vi "niScope Multi Fetch Array Measurement Cluster.vi"(0 "instrument handle":refnum<k15>, 1 "timeout":dbl=5.0 format="%.2f", 5 "channels":string="0", 7 "array measurement":T3=4000 items=["None"=4000, "Last Acq. Histogram"=4001, "Multi Acq. Voltage Histogram"=4004, "Multi Acq. Time Histogram"=4005, "Multi Acq. Average"=4016, "Polynomial Interpolation"=4011, "Array Integral"=4006, "Derivative"=4007, "Inverse"=4008, "Multiply Channels"=4012, "Add Channels"=4013, "Subtract Channels"=4014, "Divide Channels"=4015, "Array Offset"=4025, "Array Gain"=4026, "Hanning Window"=4009, "Flat Top Window"=4010, "Hamming Window"=4020, "Triangle Window"=4023, "Blackman Window"=4024, "FIR Windowed Filter"=4021, "Bessel IIR Filter"=4022, "Butterworth IIR Filter"=4017, "Chebyshev IIR Filter"=4018, "FFT Phase Spectrum"=4002, "FFT Amp. Spectrum (Volts RMS)"=4003, "FFT Amp. Spectrum (dB)"=4019], 11 "error in":errorcluster, 12 "meas waveform size":i32=-1) -> (4 "instrument handle out":refnum<k15>, 6 "wfm info":T1(array[cluster]) {"reserved2" format="%.2f"; "reserved1" format="%.2f"; "offset" format="%^.3e"; "gain" format="%^.3e"; "xIncrement" format="%^.3e"; "relativeInitialX" format="%^.3e"; "absoluteInitialX" format="%^.3e"}, 10 "meas waveform":T2(array[cluster]) {"measWfm" format="%.2f"; "xIncrement" format="%.2f"; "relativeInitialX" format="%.2f"}, 15 "error out":errorcluster)   [LabVIEW 2011]
doc: "Obtains a waveform from the digitizer and returns the specified array measurement for multiple channels and records as a cluster."
uses:
  <instrlib>/niScope/Controls/niScope array measurement.ctl
  niScope_32.dll
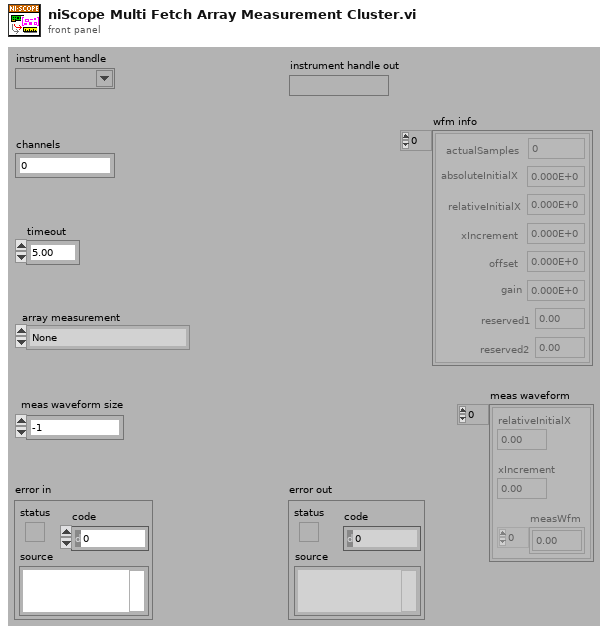
[diagram p1: front panel]
types:
  T1 = cluster{"actualSamples":i32, "absoluteInitialX":dbl, "relativeInitialX":dbl, "xIncrement":dbl, "offset":dbl, "gain":dbl, "reserved1":dbl, "reserved2":dbl}[]
  T2 = cluster{"relativeInitialX":dbl, "xIncrement":dbl, "measWfm":dbl[]}[]
  T3 = typedef "niScope array measurement.ctl" = i32
  T4 = cluster{"Element Data":i32, "Element Data":dbl, "Element Data":dbl, "Element Data":dbl, "Element Data":dbl, "Element Data":dbl, "Element Data":dbl, "Element Data":dbl}
  T5 = cluster{"Element Data":dbl, "Element Data":dbl, "measWfm":dbl[]}
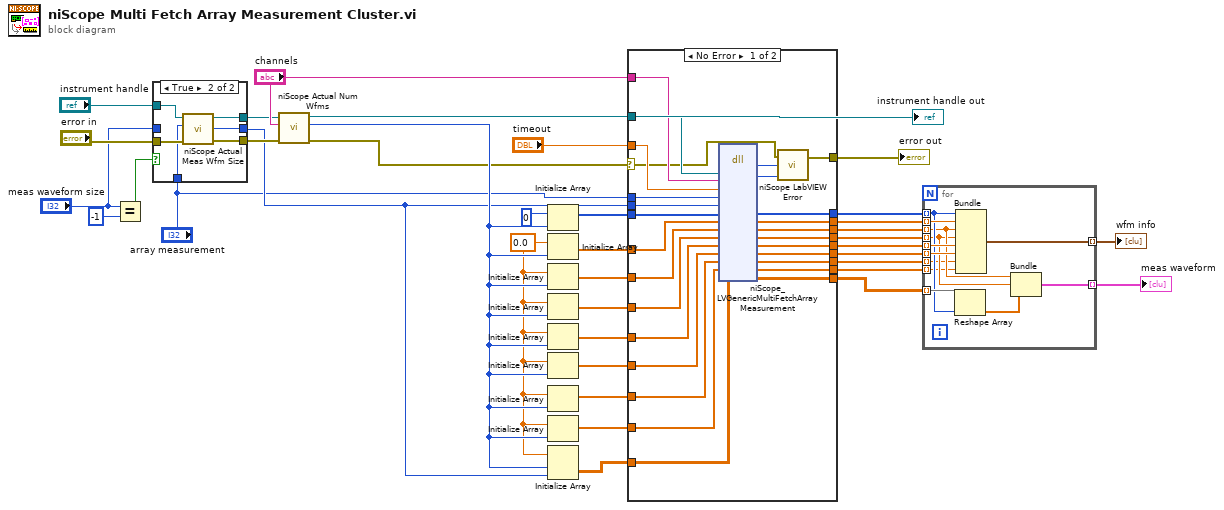
[diagram p0: block diagram]
diagram:
  w8 = 0.0 ("Element Data")
  n1 = Equal?(x="meas waveform size", y=-1) -> (x = y?=w34:bool)
  n2 = case shown="True" w34 {
    tunnel: [w40 w46] -> w33
    tunnel: "error in" -> [w40 w45]
    tunnel: "instrument handle" -> [w39 w44]
    tunnel: [w39 w43] -> w30
    tunnel: [w38 w42] -> w27
    tunnel: "meas waveform size" -> [w38 _]
    tunnel: "array measurement" -> [_ w41]
    frame False {
    }
    frame True {
      n3 = call <instrlib>:"niScope Actual Meas Wfm Size.vi"("error in"=w45, "arrayMeasFunction"=w41, "instrument handle"=w44) -> ("error out"=w46:errorcluster, "meas wfm size"=w42:i32, "instrument handle out"=w43:refnum<k15>)  [unwired: 6 in]
    }
  }
  n4 = call <instrlib>:"niScope Actual Num Wfms.vi"("error in"=w33, "channels"="channels", "instrument handle"=w30) -> ("error out"=w1:errorcluster, "actual num wfms"=w28:i32, "instrument handle out"=w26:refnum<k15>)  [unwired: 6 in]
  "instrument handle out" <- w26
  n5 = Initialize Array(0 ("Element Data"), w28) -> (w18:i32[])
  n6 = Initialize Array(w8, w28) -> (w19:dbl[])
  n7 = Initialize Array(w8, w28) -> (w2:dbl[])
  n8 = Initialize Array(w8, w28) -> (w20:dbl[])
  n9 = Initialize Array(w8, w28) -> (w21:dbl[])
  n10 = Initialize Array(w8, w28) -> (w9:dbl[])
  n11 = Initialize Array(w8, w28) -> (w7:dbl[])
  n12 = Initialize Array(w8, w28) -> (w6:dbl[])
  n13 = Initialize Array(w8, w28, w27) -> (w10:dbl[][])
  n14 = case shown="No Error" w1 {
    selector: w1 -> [w47 w74]
    tunnel: [w73 w74] -> w37
    tunnel: "channels" -> [w72 _]
    tunnel: w27 -> [w71 _]
    tunnel: w26 -> [w70 _]
    tunnel: "array measurement" -> [w69 _]
    tunnel: w21 -> [w66 w79]
    tunnel: w20 -> [w65 w80]
    tunnel: w2 -> [w64 w81]
    tunnel: w19 -> [w63 w82]
    tunnel: w18 -> [w62 w83]
    tunnel: "timeout" -> [w61 _]
    tunnel: [w60 w78] -> w16
    tunnel: [w59 w79] -> w15
    tunnel: [w58 w80] -> w14
    tunnel: [w57 w81] -> w13
    tunnel: [w56 w82] -> w12
    tunnel: [w55 w83] -> w11
    tunnel: w10 -> [w54 w75]
    tunnel: w9 -> [w53 w78]
    tunnel: w7 -> [w52 w77]
    tunnel: w6 -> [w51 w76]
    tunnel: [w50 w75] -> w5
    tunnel: [w49 w77] -> w4
    tunnel: [w48 w76] -> w3
    frame No Error {
      n15 = dll-call lib="niScope_*.*" fn="niScope_LVGenericMultiFetchArrayMeasurement"("instrument handle"=w70, "channelList"=w72, "timeout"=w61, "arrayMeasFunction"=w69, "measWfmSize"=w71, "actualSamples"=w62, "absoluteInitialX"=w63, "relativeInitialX"=w64, "xIncrement"=w65, "offset"=w66, "gain"=w53, "reserved1"=w52, "reserved2"=w51, "measWfm"=w54) -> ("status"=w68:i32, "instrument handle"=w67:u32, "actualSamples"=w55:i32[], "absoluteInitialX"=w56:dbl[], "relativeInitialX"=w57:dbl[], "xIncrement"=w58:dbl[], "offset"=w59:dbl[], "gain"=w60:dbl[], "reserved1"=w49:dbl[], "reserved2"=w48:dbl[], "measWfm"=w50:dbl[][])  [unwired: 7 in, 2 out]
      n16 = call <instrlib>:"niScope LabVIEW Error.vi"("instrument handle"=w67, "niScope error code (0)"=w68, "error in (no error)"=w47) -> ("error out"=w73:errorcluster)  [unwired: 2 in]
    }
    frame Error {
    }
  }
  "error out" <- w37
  n17 = for {
    tunnel: w11 -> [w91] mode=indexing
    tunnel: w12 -> [w95] mode=indexing
    tunnel: w13 -> [w90] mode=indexing
    tunnel: w14 -> [w89] mode=indexing
    tunnel: w15 -> [w94] mode=indexing
    tunnel: w16 -> [w93] mode=indexing
    tunnel: w5 -> [w92] mode=indexing
    tunnel: [w87] -> w24 mode=indexing
    tunnel: [w86] -> w25 mode=indexing
    tunnel: w4 -> [w85] mode=indexing
    tunnel: w3 -> [w84] mode=indexing
    n18 = Reshape Array(w92, w91) -> (w88:dbl[])
    n19 = Bundle("Element Data"=w91, "Element Data"=w95, "Element Data"=w90, "Element Data"=w89, "Element Data"=w94, "Element Data"=w93, "Element Data"=w85, "Element Data"=w84) -> (w87:T4)  [unwired: 1 in]
    n20 = Bundle("Element Data"=w90, "Element Data"=w89, "measWfm"=w88) -> (w86:T5)  [unwired: 1 in]
  }
  "meas waveform" <- w25
  "wfm info" <- w24
